vi "CLSUIP_ExcludeInInterfaceInheritance.vi"(9 "exclude these":string[](array[string]), 10 "inherited in":T1(array[cluster]), 11 "available in":T1(array[cluster])) -> (2 "inherited out":T1(array[cluster]), 3 "available out":T1(array[cluster]))   [LabVIEW 2021]
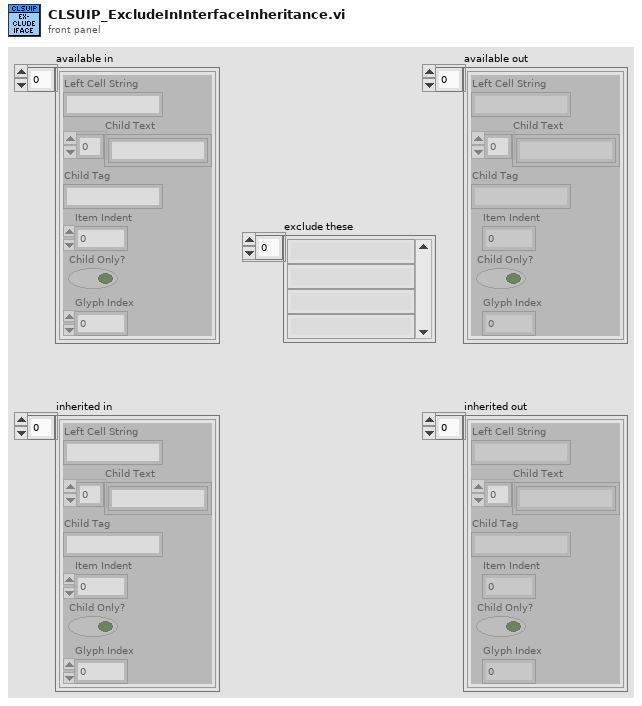
[diagram p1: front panel]
types:
  T1 = cluster{"Left Cell String":string, "Child Text":string[], "Child Tag":string, "Item Indent":i32, "Child Only?":bool, "Glyph Index":i32}[]
  T2 = cluster{"Left Cell String":string, "Child Text":string[], "Child Tag":string, "Item Indent":i32, "Child Only?":bool, "Glyph Index":i32}
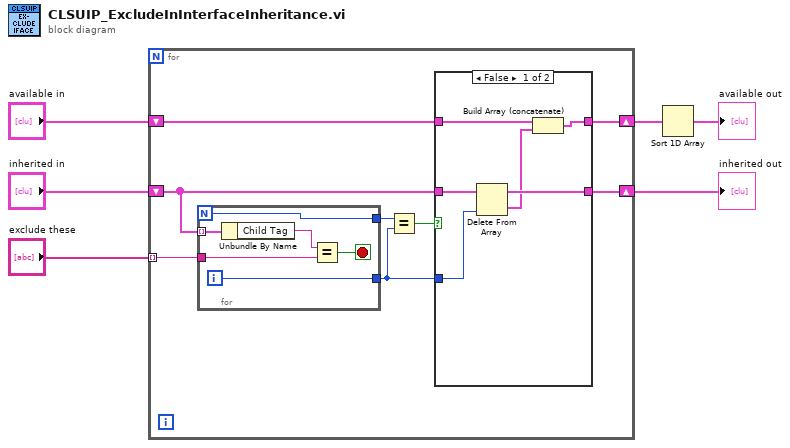
[diagram p0: block diagram]
diagram:
  n1 = for {
    tunnel: "exclude these" -> [w14] mode=indexing
    shift-right: [w11] -> w2
    shift-left: "available in" -> [w10]
    shift-right: [w9] -> w3
    shift-left: "inherited in" -> [w8]
    n2 = for {
      N -> [w23]
      tunnel: w8 -> [w28] mode=indexing
      tunnel: w14 -> [w26]
      tunnel: [w24] -> w7
      tunnel: [w23] -> w13
      i -> [w24]
      stop <- w25 stop-if-true
      n3 = Unbundle By Name(w28) -> ("Child Tag"=w27:string)
      n4 = Equal?(x=w27, y=w26) -> (x = y?=w25:bool)
    }
    n5 = Equal?(x=w13, y=w7) -> (x = y?=w12:bool)
    n6 = case shown="False" w12 {
      tunnel: [w16 w22] -> w11
      tunnel: w10 -> [w17 w22]
      tunnel: [w18 w21] -> w9
      tunnel: w8 -> [w20 w21]
      tunnel: w7 -> [w19 _]
      frame False {
        n7 = Delete From Array(array=w20, index=w19) -> (deleted portion=w15:T2, array with subset deleted=w18:T1)  [unwired: 1 in]
        n8 = Build Array (concatenate)(w17, w15) -> (w16:T1)
      }
      frame True {
        # "Not found."
      }
    }
  }
  "inherited out" <- w3
  n9 = Sort 1D Array(array=w2) -> (sorted array=→"available out":T1)
